vi "Draw_3D_Box.vi"(1 "Box Coordinates":cluster{"Max":dbl, "Min":dbl}[](array[cluster])=[{"Max"=16000.0, "Min"=14000.0}, {"Max"=1000.0, "Min"=-1000.0}, {"Max"=700.0, "Min"=0.0}] {"Min" format="%.1f"; "Max" format="%.1f"}, 2 "Name":string, 3 "Color":T1={"Red"=1.0, "Green"=0.0, "Blue"=0.0, "Alpha"=1.0}) -> (0 "Translated Object":refnum<vi>)   [LabVIEW 2013]
uses:
  <vilib>/picture/3D Picture Control/Object/Create Object (name).vi
  <vilib>/picture/3D Picture Control/NI_3D Picture Control.lvlib
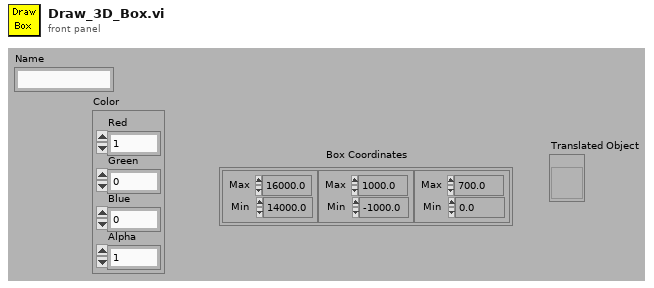
[diagram p1: front panel]
types:
  T1 = cluster{"Red":sgl, "Green":sgl, "Blue":sgl, "Alpha":sgl}
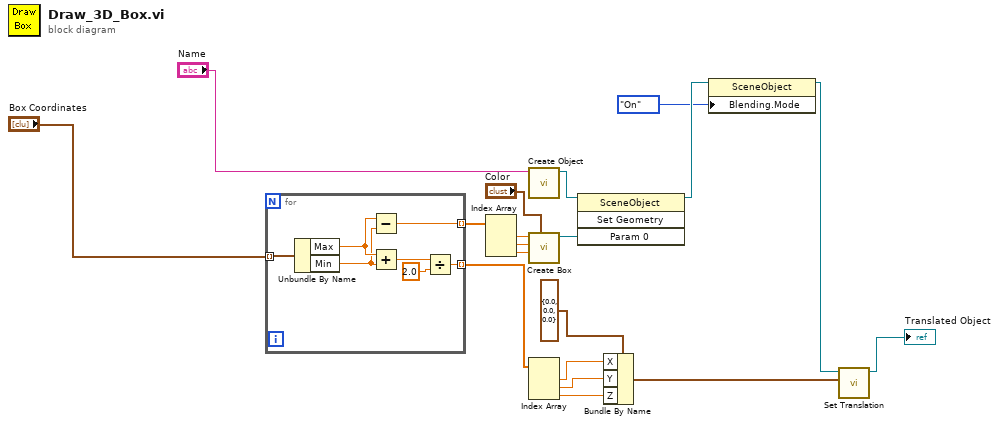
[diagram p0: block diagram]
diagram:
  n1 = for {
    tunnel: "Box Coordinates" -> [w26] mode=indexing
    tunnel: [w25] -> w18 mode=indexing
    tunnel: [w22] -> w13 mode=indexing
    n2 = Unbundle By Name(w26) -> ("Max"=w21:dbl, "Min"=w20:dbl)
    n3 = Subtract(x=w21, y=w20) -> (x-y=w25:dbl)
    n4 = Add(x=w21, y=w20) -> (x+y=w24:dbl)
    n5 = Divide(x=w24, y=2.0) -> (x/y=w22:dbl)
  }
  n6 = Index Array(array=w18) -> (element #1=w17:dbl, element #2=w16:dbl, element #3=w15:dbl)  [unwired: 3 in]
  n7 = call-poly <vilib>:"Create Object.vi"("Name"="Name") -> ("Scene:New Object"=w5:refnum<vi>)  [unwired: 9 in, 1 out]
  n8 = call <vilib>:"Create Box.vi"("Color 2"="Color", "Length Z"=w15, "Length Y"=w16, "Length X"=w17) -> ("New Box Refnum"=w8:refnum<vi>)  [unwired: 6 in, 1 out]
  n9 = Index Array(array=w13) -> (element #1=w12:dbl, element #2=w11:dbl, element #3=w10:dbl)  [unwired: 3 in]
  n10 = invoke class="SceneObject" method="Set Geometry"(reference=w5, "Param 0"=w8) -> (reference out=w3:refnum<vi>)  [unwired: 2 in, 3 out]
  n11 = Bundle By Name(cluster=cluster{"X":sgl, "Y":sgl, "Z":sgl} {"X"=0.0, "Y"=0.0, "Z"=0.0} ("Translation"), "X"=w12, "Y"=w11, "Z"=w10) -> (w9:cluster{"X":sgl, "Y":sgl, "Z":sgl})
  n12 = property class="SceneObject"(reference=w3, "Blending.Mode"=enum16{"Inherit Value", "Off", "On"}."On" ("Blending:Mode")) -> (reference out=w2:refnum<vi>)  [unwired: 1 in, 1 out]
  n13 = call <vilib>:"Set Translation.vi"("Translation"=w9, "Scene Object"=w2) -> ("Translated Object"=→"Translated Object":refnum<vi>)  [unwired: 8 in, 1 out]
